vi "MHM Save Register.vi"(6 "pulData":u32[](array[numeric]), 7 "pulNumerOfBytes":u32, 8 "error in (no error)":errorcluster, 9 "ulAdr":u32, 10 "pcFilename":string, 11 "ulMHMHandle":u32) -> (0 "error out":errorcluster, 3 "function return":u32)   [LabVIEW 2017, in "MHM_1SL_interface.lvlib"]
uses:
  MHM_1SL_interface.lvlib
  SSI_Tool/DUT_Interface/lv_interface/lib/MHM_1SL_interface.dll
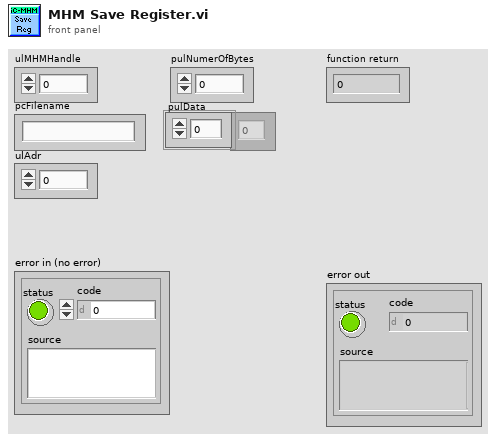
[diagram p1: front panel]
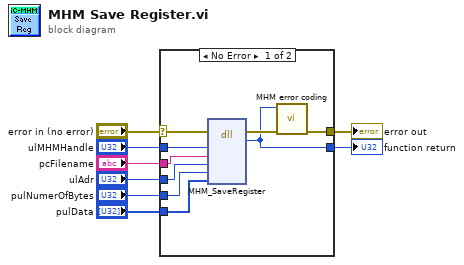
[diagram p0: block diagram]
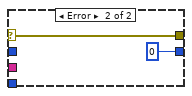
[diagram p2: hidden frame]
diagram:
  n1 = case shown="No Error" "error in (no error)" {
    selector: "error in (no error)" -> [w17 w19]
    tunnel: "ulMHMHandle" -> [w16 _]
    tunnel: [w14 w19] -> w7
    tunnel: [w13 u32 0 ("return type")] -> w8
    tunnel: "pcFilename" -> [w12 _]
    tunnel: "ulAdr" -> [w11 _]
    tunnel: "pulNumerOfBytes" -> [w10 _]
    tunnel: "pulData" -> [w9 _]
    frame No Error {
      n2 = dll-call lib="C:/workspace/project/scancon/sw/SSI_Tool/DUT_Interface/lv_interface/lib/MHM_1SL_interface.dll" fn="MHM_SaveRegister"(error in=w17, "ulMHMHandle"=w16, "pcFilename"=w12, "ulAdr"=w11, "pulNumerOfBytes"=w10, "pulData"=w9) -> (error out=w15:errorcluster, "return type"=w13:u32)  [unwired: 7 in, 1 out]
      n3 = call "MHM error coding.vi"("error in (no error)"=w15, "function return in"=w13) -> ("error out"=w14:errorcluster)  [unwired: 9 in]
    }
    frame Error {
    }
  }
  "function return" <- w8
  "error out" <- w7
